vi "Maestro.vi"() -> ()   [LabVIEW 2017]
uses:
  Enum_1.ctl
  <vilib>/Modbus/master/Modbus Master.lvclass
  <vilib>/Modbus/master/Create Master Instance (TCP).vi
  <vilib>/addons/_office/excel.llb/Excel Get Data (dbl).vi
  <vilib>/addons/_office/excel.llb/Excel Easy Table (num).vi
  <vilib>/Utility/NIReport.llb/NI_report.lvclass
  <vilib>/addons/_office/NI_ReportGenerationToolkit.lvlib
  <vilib>/Utility/NIReport.llb/Excel/NI_Excel.lvclass
panel:
  in  "stop":bool
  in  "coil values":bool[](array[boolean])
  in  "holding register values":u16[](array[numeric])
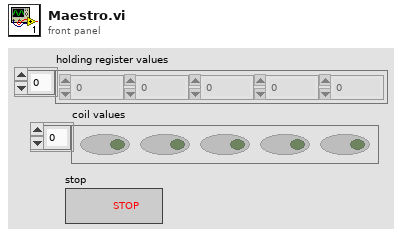
[diagram p1: front panel]
types:
  T1 = cluster{"TCP master instance":refnum<class "Modbus Master.lvclass">, "error in (no error)":errorcluster, "Ruta del Reporte":path, "Registro":i32}
  T2 = typedef "Enum_1.ctl" = enum16{"Configuracion", "Espera", "Actualizar Reporte"}
  T3 = enum16{"Standard Report", "HTML", "Word", "Excel"}
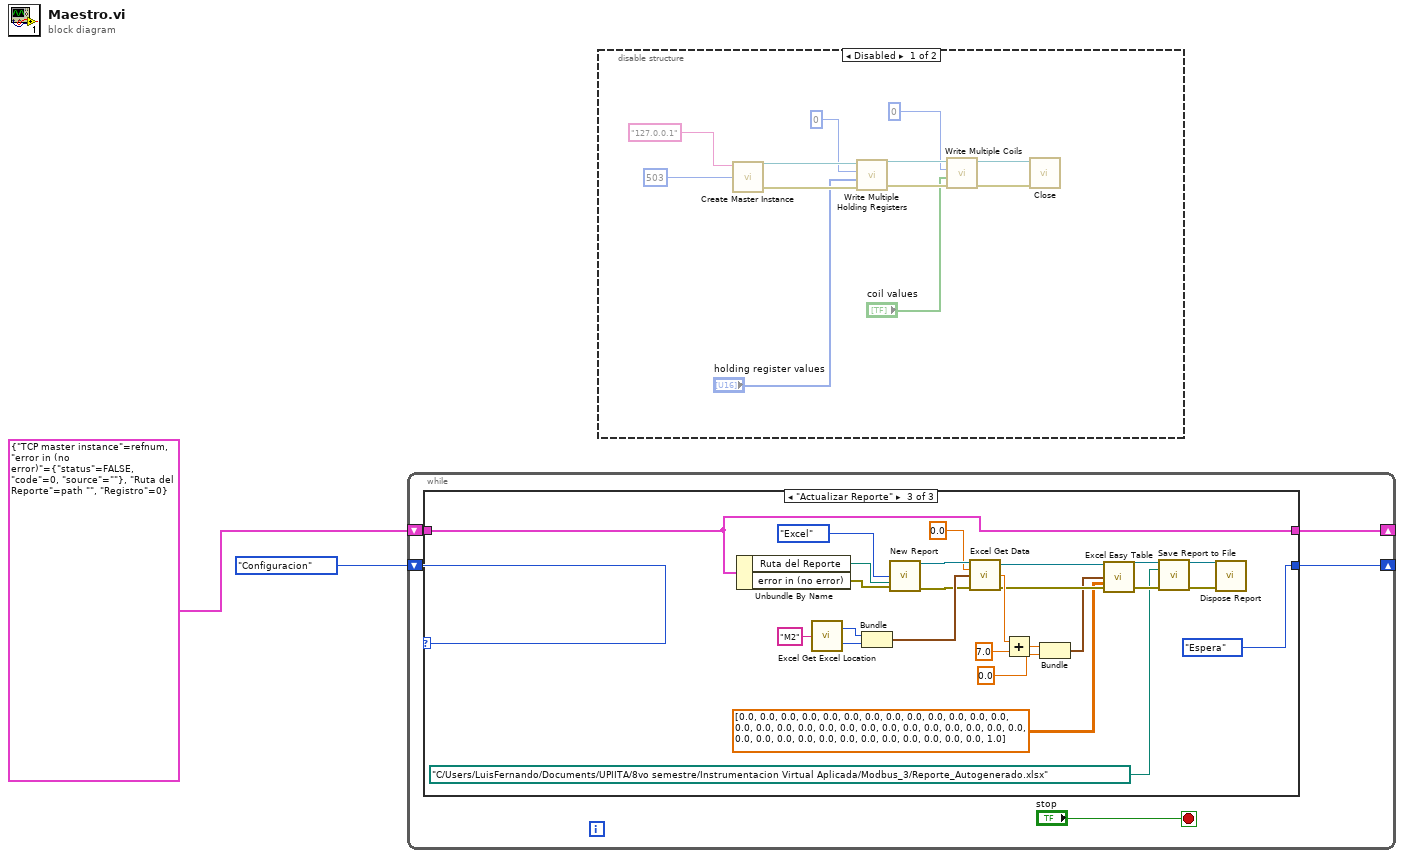
[diagram p0: block diagram]
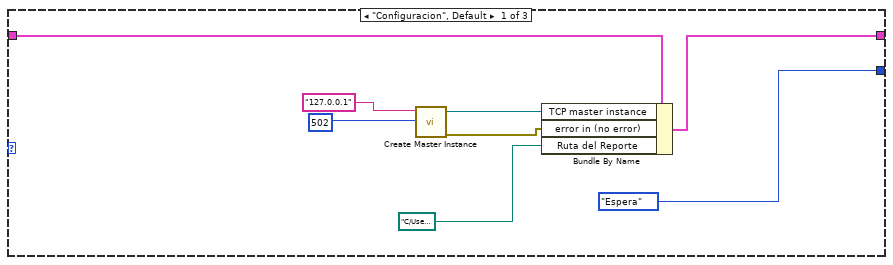
[diagram p2: hidden frame]
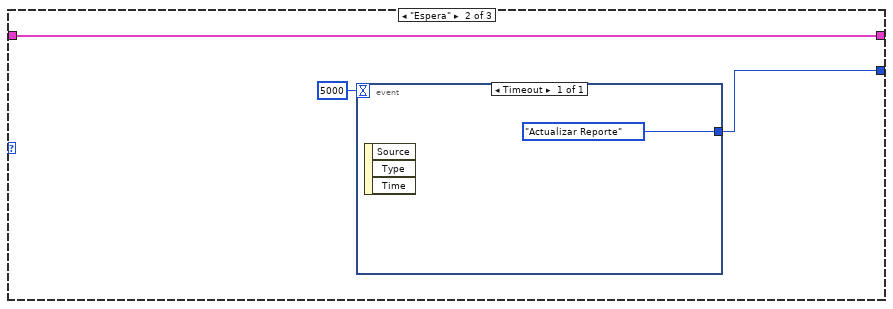
[diagram p3: hidden frame]
diagram:
  n1 = while {
    shift-right: [w3] -> _
    shift-left: Enum_1."Configuracion" -> [w7]
    shift-right: [w5] -> _
    shift-left: T1 {"TCP master instance"=refnum, "error in (no error)"={"status"=FALSE, "code"=0, "source"=""}, "Ruta del Reporte"=path "", "Registro"=0} -> [w6]
    stop <- "stop" stop-if-true
    n2 = case shown="\"Actualizar Reporte\"" w7 {
      tunnel: w6 -> [w13 w18 w20]
      tunnel: [w12 w18 w20] -> w5
      tunnel: [Enum_1."Espera" w16 Enum_1."Espera"] -> w3
      frame "Configuracion", Default {
        n3 = call-poly <vilib>:"Create Master Instance.vi"("port (502)"=u16 502, "address"="127.0.0.1") -> ("error out"=w10:errorcluster, "TCP master instance"=w11:refnum<class "Modbus Master.lvclass">)  [unwired: 8 in]
        n4 = Bundle By Name(cluster=w13, "TCP master instance"=w11, "error in (no error)"=w10, "Ruta del Reporte"=path "C:/Users/LuisFernando/Documents/UPIITA/8vo semestre/Instrumentacion Virtual Aplicada/Modbus_3") -> (w12:T1)
      }
      frame "Espera" {
        n5 = event shown="[0] Timeout" {
          selector: _ -> [_]
          dyn-events: _ -> [_]
          timeout: 5000 -> [_]
          tunnel: [Enum_1."Actualizar Reporte"] -> w16
          event Timeout {
            n6 = event-data() -> ()  [unwired: 1 in, 3 out]
          }
        }
      }
      frame "Actualizar Reporte" {
        n7 = Unbundle By Name(w20) -> ("Ruta del Reporte"=w43:path, "error in (no error)"=w36:errorcluster)
        n8 = call <vilib>:"Excel Get Excel Location.vi"("cell's name"="M2") -> ("row"=w40:i32, "column"=w39:i32)
        n9 = Bundle("row"=w40, "column"=w39) -> (w38:cluster{"row":i32, "column":i32})  [unwired: 1 in]
        n10 = call <vilib>:"New Report.vi"("report type"=T3."Excel", "template (empty)"=w43, "error in (no error)"=w36) -> ("report out"=w42:refnum<class "NI_report.lvclass">, "error out"=w37:errorcluster)  [unwired: 11 in]
        n11 = call-poly <vilib>:"Excel Get Data.vi"("report in"=w42, "data type"=0.0, "start (0, 0)"=w38, "error in (no error)"=w37) -> ("report out"=w30:refnum<class "NI_report.lvclass">, "data"=w34:dbl, "error out"=w29:errorcluster)  [unwired: 9 in]
        n12 = Add(x=w34, y=7.0) -> (x+y=w32:dbl)
        n13 = Bundle(w32, 0.0) -> (w28:cluster{dbl, dbl})  [unwired: 1 in]
        n14 = call-poly <vilib>:"Excel Easy Table.vi"("report in"=w30, "start (0, 0)"=w28, "text data"=dbl[][] [[0.0, 0.0, 0.0, 0.0, 0.0, 0.0, 0.0, 0.0, 0.0, 0.0, 0.0, 0.0, 0.0, 0.0, 0.0, 0.0, 0.0, 0.0, 0.0, 0.0], [0.0, 0.0, 0.0, 0.0, 0.0, 0.0, 0.0, 0.0, 0.0, 0.0, 0.0, 0.0, 0.0, 0.0, 0.0, 0.0, 0.0, 0.0, 0.0, 1.0]], "error in (no error)"=w29) -> ("report out"=w25:refnum<class "NI_report.lvclass">, "error out"=w26:errorcluster)  [unwired: 7 in, 3 out]
        n15 = call-dynamic "Save Report to File.vi"("report in"=w25, "report file path"=path "C:/Users/LuisFernando/Documents/UPIITA/8vo semestre/Instrumentacion Virtual Aplicada/Modbus_3/Reporte_Autogenerado.xlsx", "error in (no error)"=w26) -> ("report out"=w24:refnum<class "NI_report.lvclass">, "error out"=w23:errorcluster)  [unwired: 11 in]
        n16 = call-dynamic "Dispose Report.vi"("report in"=w24, "error in (no error)"=w23) -> ()  [unwired: 13 in, 1 out]
      }
    }
  }
  n17 = disable-structure shown="Disabled" {
    frame Disabled {
      n18 = call-poly <vilib>:"Create Master Instance.vi"("port (502)"=u16 503, "address"="127.0.0.1") -> ("error out"=w55:errorcluster, "TCP master instance"=w56:refnum<class "Modbus Master.lvclass">)  [unwired: 8 in]
      n19 = call-dynamic "Write Multiple Holding Registers.vi"("error in (no error)"=w55, "holding register values"="holding register values", "starting address"=u16 0, "Modbus master in"=w56) -> ("error out"=w49:errorcluster, "Modbus master out"=w50:refnum<class "Modbus Master.lvclass">)  [unwired: 6 in]
      n20 = call-dynamic "Write Multiple Coils.vi"("error in (no error)"=w49, "coil values"="coil values", "starting address"=u16 0, "Modbus master in"=w50) -> ("error out"=w46:errorcluster, "Modbus master out"=w45:refnum<class "Modbus Master.lvclass">)  [unwired: 6 in]
      n21 = call-dynamic "Close.vi"("error in (no error)"=w46, "Modbus master in"=w45) -> ()  [unwired: 9 in, 1 out]
    }
    frame Enabled {
    }
  }
